vi "InsertOneError.vi"(4 "Description":string, 6 "Library":string, 8 "ErrorIn":errorcluster caption="Error In(no Error)", 9 "Text":string, 10 "ErrorCode":i32, 11 "ReferenceIn":refnum<class "ErrorDefinitionSQLite.lvclass"> caption="Reference In") -> (0 "ErrorOut":errorcluster caption="Error Out", 3 "ReferenceOut":refnum<class "ErrorDefinitionSQLite.lvclass"> caption="Reference Out")   [LabVIEW 2021, in "ErrorDefinitionSQLite.lvclass"]
uses:
  ErrorDefinitionSQLite.lvclass
  <vilib>/drjdpowell/SQLite Library/SQL Connection/Execute SQL.vi
  <vilib>/drjdpowell/SQLite Library/SQLite.lvlib
  <vilib>/drjdpowell/SQLite Library/SQL Connection/Connection.lvclass
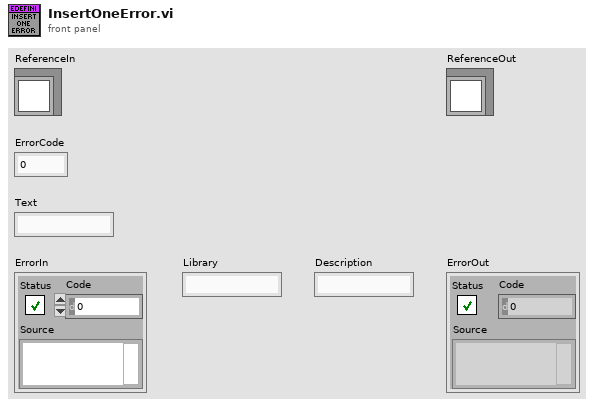
[diagram p1: front panel]
types:
  T1 = typedef "ErrorDefinitionSQLite.lvclass/ObjectAttributes.ctl" = cluster{"Path":path, "SQLiteRef":refnum<class "Connection.lvclass">, "EndOfRange":i32, "DefaultLibrarySize":i32, "StartOfRange":i32}
  T2 = cluster{string, "Text":string, "Library":string, "Description":string, "App.UserName":string}
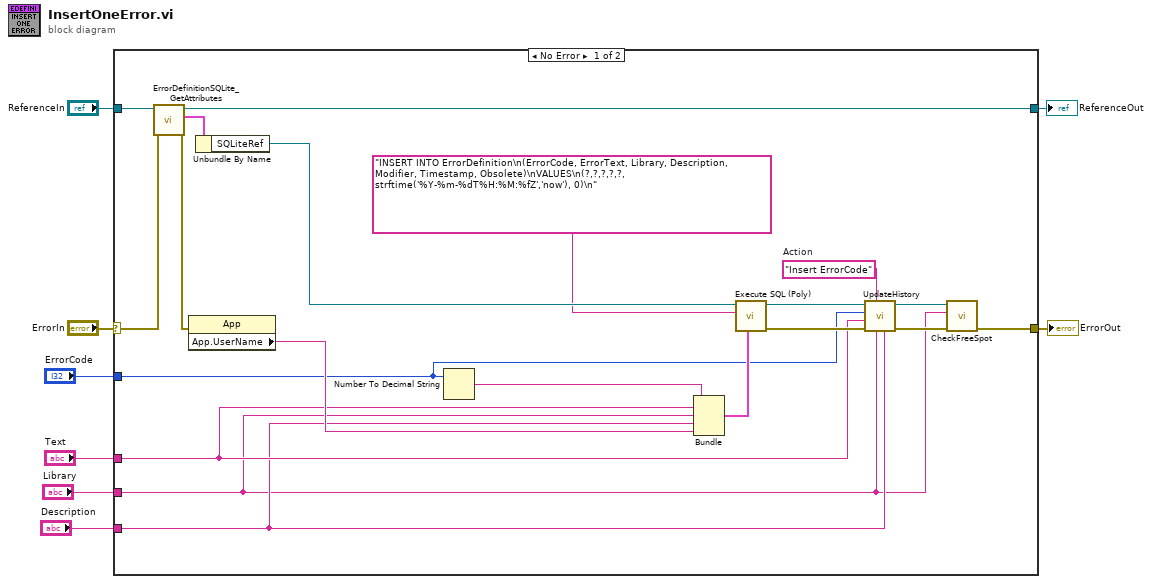
[diagram p0: block diagram]
diagram:
  n1 = case shown="No Error" "ErrorIn" {
    selector: "ErrorIn" -> [w28 w30]
    tunnel: [w10 w30] -> w7
    tunnel: [w26 w29] -> w5
    tunnel: "ReferenceIn" -> [w27 w29]
    tunnel: "ErrorCode" -> [w15 _]
    tunnel: "Text" -> [w14 _]
    tunnel: "Library" -> [w9 _]
    tunnel: "Description" -> [w13 _]
    frame No Error {
      w23 = "Insert ErrorCode"  # Action
      n2 = call "ErrorDefinitionSQLite_GetAttributes.vi"("ErrorIn"=w28, "Reference in"=w27) -> ("ErrorOut"=w20:errorcluster, "Data"=w25:T1, "Reference out"=w26:refnum<class "ErrorDefinitionSQLite.lvclass">)  [unwired: 6 in, 1 out]
      n3 = property class="App"(error in=w20) -> ("App.UserName"=w19:string)  [unwired: 1 in, 2 out]
      n4 = Unbundle By Name(w25) -> ("SQLiteRef"=w18:refnum<class "Connection.lvclass">)
      n5 = Number To Decimal String(number=w15) -> (decimal integer string=w16:string)  [unwired: 1 in]
      n6 = Bundle(w16, "Text"=w14, "Library"=w9, "Description"=w13, "App.UserName"=w19) -> (w24:T2)  [unwired: 1 in]
      n7 = call-poly <vilib>:"Execute SQL (Poly).vi"("Parameter(s)"=w24, "SQL"="INSERT INTO ErrorDefinition\n(ErrorCode, ErrorText, Library, Description, Modifier, Timestamp, Obsolete)\nVALUES\n(?,?,?,?,?, strftime('%Y-%m-%dT%H:%M:%fZ','now'), 0)\n", "SQLite Connection in"=w18) -> ("error out"=w21:errorcluster, "SQLite Connection"=w22:refnum<class "Connection.lvclass">)  [unwired: 5 in, 2 out]
      n8 = call "UpdateHistory.vi"("Description"=w13, "Library"=w9, "Action"=w23, "error in (no error)"=w21, "ErrorText"=w14, "ErrorCode"=w15, "Connection in"=w22) -> ("error out"=w12:errorcluster, "Connection out"=w11:refnum<class "Connection.lvclass">)  [unwired: 3 in]
      n9 = call "CheckFreeSpot.vi"("error in (no error)"=w12, "LibraryName"=w9, "Connection in"=w11) -> ("error out"=w10:errorcluster)  [unwired: 4 in, 4 out]
    }
    frame Error {
    }
  }
  "ErrorOut" <- w7
  "ReferenceOut" <- w5
